vi "PH_SSAC.ProcPeriodic.vi"(0 "i ref in":refnum<vi>, 3 "ms timeout (10000)":i32=10000, 5 "error in (no error)":errorcluster) -> (14 "i ref out":refnum<vi>, 17 "timed out":bool, 19 "error out":errorcluster)   [LabVIEW 2014, in "PH_SSAC.lvlib"]
doc: "This method serves to periodically do things like reading values from the HW. Methods that should be executed periodically should be called from THIS methode. Add code here."
uses:
  PH_SSAC.lvlib
  PH_StatusHandler/PH_StatusHandler.Status.ctl
  PH_Common/PH_Common.lvlib
  PH_StatusHandler/PH_StatusHandler.lvlib
  PH_Img_BaseClass/PH_Img_BaseClass.lvlib
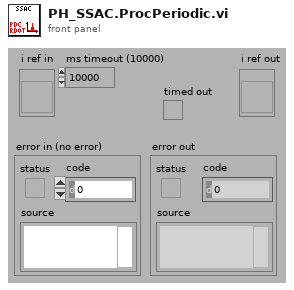
[diagram p1: front panel]
types:
  T1 = typedef "PH_SSAC.lvlib/PH_SSAC.i attribute.ctl" = cluster{"GUI Refs":cluster{"Delete":refnum<vi>, "Global On":refnum<vi>, "Cam Source":refnum<vi>, "Frame Main Signal":refnum<vi>, "Frame Background":refnum<vi>, "dt (Gauss smooth)":refnum<vi>, "Calibration Factor":refnum<vi>, "Background acquire":refnum<vi>, "Threshold":refnum<vi>, "Time evolution of mean pulse duration":refnum<vi>, "Mean Pulse Duration":refnum<vi>, "Main signal":refnum<vi>, "Current Pulse Duration":refnum<vi>, "Processed":refnum<vi>, "Saturation":refnum<vi>, "# for Average":refnum<vi>, "Position":refnum<vi>, "BG Status":refnum<vi>, "Save BG data":refnum<vi>, "Read BG Data":refnum<vi>, "Background Calibration Data":refnum<vi>}, "Images":cluster{"OP Image":T2, "GUI Image":T2, "PSDB Image":T2}, "Global On?":bool, "Frame Main":cluster{"x":u32, "dx":u32, "y":u32, "dy":u32}, "Frame Background":cluster{"x":u32, "dx":u32, "y":u32, "dy":u32}, "dt [fs]":dbl, "Calibration Factor [fs/pixel]":dbl, "Threshold":dbl, "Time evolution of mean pulse duration [fs]":dbl[], "Main Signal":cluster{"Time for Main":dbl[], "Signal":dbl[]}, "Processed":bool, "Current Pulse Duration [fs]":dbl, "# for Average":i32, "Position":i32, "Pulse Durations [fs]":dbl[], "BG":cluster{"Acquire?":bool, "Background Calibration Data":T3, "Save Data":bool}}
  T2 = typedef "IMAQ Image.ctl" = refnum<image>
  T3 = typedef "PH_SSAC.lvlib/PH_SSAC.Background Data.ctl" = cluster{"Date":string, "Time":string, "Frame Main":cluster{"x":u32, "dx":u32, "y":u32, "dy":u32}, "dt [fs]":dbl, "Calibration Factor [fs/pixel]":dbl, "Signal":dbl[], "Frame Background":cluster{"x":u32, "dx":u32, "y":u32, "dy":u32}}
  T4 = typedef "PH_StatusHandler.lvlib/PH_StatusHandler.Status.ctl" = i16
  T5 = typedef "PH_Img_BaseClass.lvlib/PH_Img_BaseClass.i attribute.ctl" = cluster{"GUI Refs":T6, "Timeout Image [ms]":i32, "Default Periodic Period [ms]":i32, "Camera":cluster{"Instancename":string, "Notifier":refnum<notifier>}, "Palette":T7, "Cam Settings":cluster{"Cam ID":string, "Gain":dbl, "Brightness":dbl, "Shutter":dbl, "Cam Info Failure":bool, "Mode":i32}}
  T6 = typedef "PH_Img_BaseClass.lvlib/PH_Img_BaseClass.GUI Refs.ctl" = cluster{"Timeout":refnum<vi>, "Image":refnum<vi>, "Palette":refnum<vi>, "Timeout Set":refnum<vi>}
  T7 = typedef "PH_Img_BaseClass.lvlib/PH_Img_BaseClass.Palette.ctl" = i32
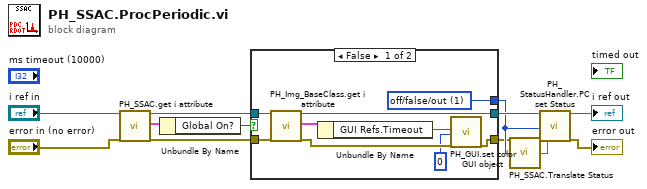
[diagram p0: block diagram]
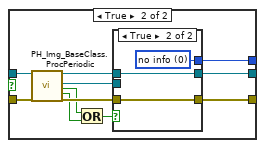
[diagram p2: hidden frame]
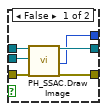
[diagram p3: hidden frame]
diagram:
  n1 = call "PH_SSAC.get i attribute.vi"("i ref in"="i ref in", "error in (no error)"="error in (no error)") -> ("i ref out"=w11:refnum<vi>, "i attribute"=w12:T1, "error out"=w10:errorcluster)  [unwired: 15 in]
  n2 = Unbundle By Name(w12) -> ("Global On?"=w6:bool)
  n3 = case shown="False" w6 {
    tunnel: [w14 w32] -> w2
    tunnel: w11 -> [w21 w27]
    tunnel: w10 -> [w18 w29]
    tunnel: [w19 w31] -> w8
    tunnel: [w20 w30] -> w3
    frame False {
      w20 = T4 1 items=["no info", "off/false/out", "on/true/in", "Failure", "Alarm", "Status 1", "Status 2", "Status 3"] ("Status.Device Status")
      n4 = call "PH_Img_BaseClass.get i attribute.vi"("i ref in"=w21, "error in (no error)"=w18) -> ("i ref out"=w19:refnum<vi>, "i attribute"=w17:T5, "error out"=w15:errorcluster)  [unwired: 15 in]
      n5 = Unbundle By Name(w17) -> ("GUI Refs.Timeout"=w16:refnum<vi>)
      n6 = call "PH_GUI.set color GUI object.vi"("GUI object Ref"=w16, "State"=0, "error in (no error)"=w15) -> ("error out"=w14:errorcluster)  [unwired: 16 in]
    }
    frame True {
      n7 = call "PH_Img_BaseClass.ProcPeriodic.vi"("i ref in"=w27, "error in (no error)"=w29) -> ("i ref out"=w26:refnum<vi>, "Cam Image"=w25:T2, "timed out?"=w23:bool, "Error while unflatten data?"=w22:bool, "error out"=w28:errorcluster)  [unwired: 13 in]
      n8 = Or(x=w23, y=w22) -> (x .or. y?=w24:bool)
      n9 = case shown="True" w24 {
        tunnel: w26 -> [w38 w41]
        tunnel: [w35 w41] -> w31
        tunnel: w28 -> [w37 w40]
        tunnel: [w36 w40] -> w32
        tunnel: w25 -> [w33 _]
        tunnel: [w34 w39] -> w30
        frame False {
          n10 = call "PH_SSAC.Draw Image.vi"("i ref in"=w38, "Image"=w33, "error in (no error)"=w37) -> ("i ref out"=w35:refnum<vi>, "Status"=w34:T4, "error out"=w36:errorcluster)  [unwired: 14 in]
        }
        frame True {
          w39 = T4 0 items=["no info", "off/false/out", "on/true/in", "Failure", "Alarm", "Status 1", "Status 2", "Status 3"] ("Status.Device Status")
        }
      }
    }
  }
  n11 = call "PH_SSAC.Translate Status.vi"("Device Status"=w3) -> ("Translated Status"=w1:string)
  n12 = call "PH_StatusHandler.PC set Status.vi"("i ref in"=w8, "Status"=w3, "error in (no error)"=w2, "Tip Strip"=w1) -> ("i ref out"=→"i ref out":refnum<vi>, "error out"=→"error out":errorcluster)  [unwired: 14 in]
